vi "Clase8b.vi"() -> ()   [LabVIEW 2013]
panel:
  out "Contador":dbl
  out "Numero 50-100":dbl
  # "Generar 10 numero entre 50-150, usar un ciclo while para validar que el numero se \nencuentre en ese rango antes de presentarlos.\nIr contando los numeros."
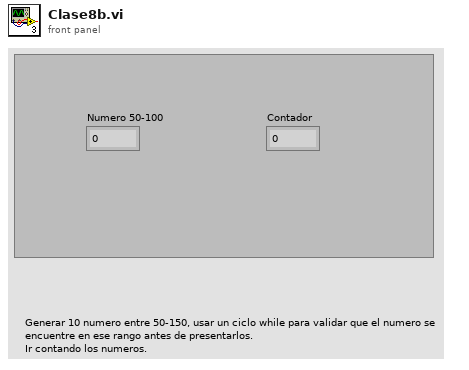
[diagram p1: front panel]
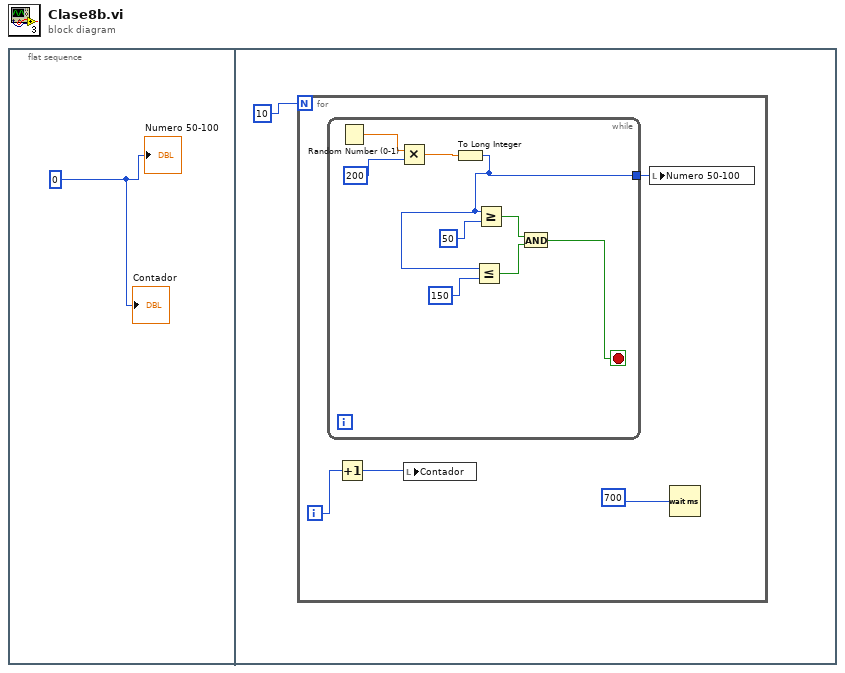
[diagram p0: block diagram]
diagram:
  n1 = flat-sequence {
    frame #0 {
      w1 = 0
      "Numero 50-100" <- w1
      "Contador" <- w1
    }
    frame #1 {
      n2 = for {
        N: 10 -> [_]
        i -> [w6]
        n3 = while {
          tunnel: [w11] -> w4
          stop <- w7 stop-if-true
          n4 = Random Number (0-1)() -> (number: 0 to 1=w15:dbl)
          n5 = Multiply(x=w15, y=200) -> (x*y=w13:dbl)
          n6 = To Long Integer(number=w13) -> (32bit integer=w11:i32)
          n7 = Less Or Equal?(x=w11, y=150) -> (x <= y?=w8:bool)
          n8 = Greater Or Equal?(x=w11, y=50) -> (x >= y?=w9:bool)
          n9 = And(x=w9, y=w8) -> (x .and. y?=w7:bool)
        }
        n10 = Increment(x=w6) -> (x+1=w5:i32)
        n11 = local write "Contador"(w5) -> ()
        n12 = local write "Numero 50-100"(w4) -> ()
        n13 = Wait (ms)(milliseconds to wait=700) -> ()  [unwired: 1 out]
      }
    }
  }
